vi "cluster_v11.vi"() -> ()   [LabVIEW 2009]
panel:
  in  "stop":bool
  in  "Delta t":dbl(slide)=5.117056856187291 scale=0.0..10.0
  out "Waveform Graph":cluster{"Slide":i32, "Slide 2":dbl, u16[]}(graph)={"Slide"=2, "Slide 2"=5.117056856187291, [11, 12, 13, 24, 15, 56, 22, 13, 0, 44, 17, 67, 42, 100, 32, 34, 55]}
  in  "to":i32(slide)=2 scale=0.0..10.0
  out "Array":dbl[](array[numeric])=[11.0, 12.0, 13.0, 24.0, 15.0, 56.0, 22.0, 13.0, 0.0, 44.0, 17.0, 67.0, 42.0, 100.0, 32.0, 34.0, 55.0]
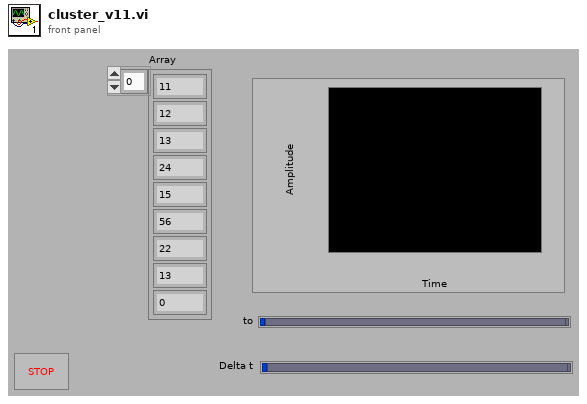
[diagram p1: front panel]
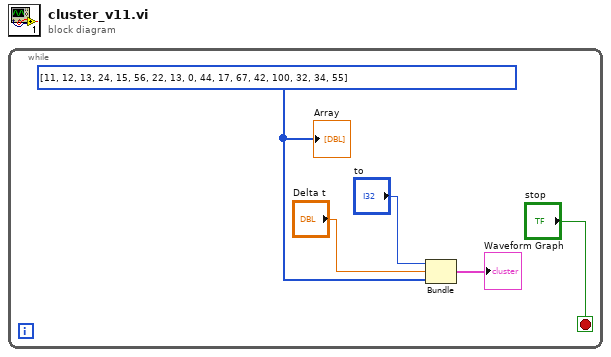
[diagram p0: block diagram]
diagram:
  n1 = while {
    stop <- "stop" stop-if-true
    w5 = u16[] [11, 12, 13, 24, 15, 56, 22, 13, 0, 44, 17, 67, 42, 100, 32, 34, 55]
    n2 = Bundle("to"="to", "Delta t"="Delta t", w5) -> (→"Waveform Graph":cluster{"to":i32, "Delta t":dbl, u16[]})  [unwired: 1 in]
    "Array" <- w5
  }
